vi "CreateLocalVI.vi"(10 "Name":string, 11 "YActor in":refnum<class "YActor.lvclass">) -> (3 "YActor out":refnum<class "YActor.lvclass">, 5 "CreatedVI":refnum<vi>)   [LabVIEW 2021, in "YActor.lvclass"]
uses:
  YActor.lvclass
  InlineReferencePool.ctl
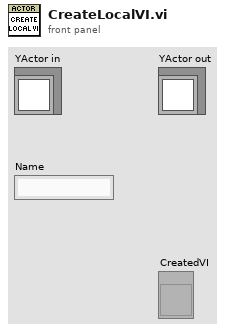
[diagram p1: front panel]
types:
  T1 = typedef "YActor.lvclass/InlineReferencePool.ctl" = enum16{"Add", "ClearAll?"}
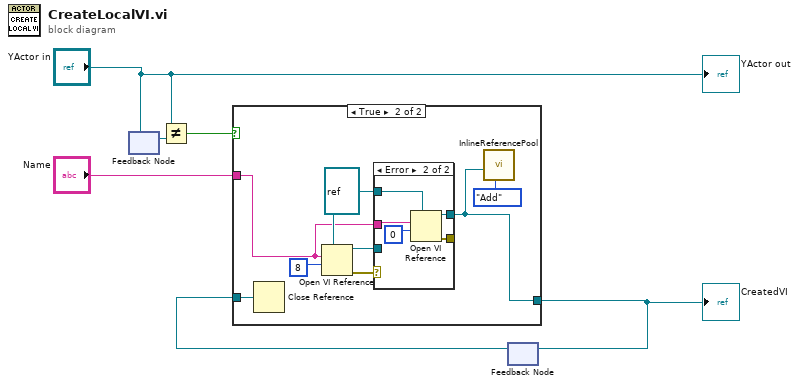
[diagram p0: block diagram]
diagram:
  n1 = feedback #1() -> (w5:refnum<class "YActor.lvclass">)  [unwired: 1 in]
  n2 = feedback-in #1("YActor in") -> ()
  n3 = Not Equal?(x="YActor in", y=w5) -> (x != y?=w6:bool)
  n4 = feedback #2() -> (w4:refnum<vi>)  [unwired: 1 in]
  n5 = case shown="True" w6 {
    tunnel: [w7 w9] -> w2
    tunnel: w4 -> [w7 w8]
    tunnel: "Name" -> [_ w11]
    frame False {
    }
    frame True {
      w14 = refnum<vi> refnum ("type specifier VI Refnum (for type only)")
      n6 = Close Reference(reference=w8) -> ()  [unwired: 1 in, 1 out]
      n7 = Open VI Reference(type specifier VI Refnum (for type only)=w14, vi path=w11, options=8) -> (vi reference=w13:refnum<vi>, error out=w15:errorcluster)  [unwired: 3 in]
      n8 = case shown="Error" w15 {
        selector: w15 -> [w17 _]
        tunnel: w11 -> [_ w21]
        tunnel: w14 -> [_ w20]
        tunnel: [w16 w19] -> w9
        tunnel: [w17 w22] -> _
        tunnel: w13 -> [w16 _]
        frame No Error {
        }
        frame Error {
          n9 = Open VI Reference(type specifier VI Refnum (for type only)=w20, vi path=w21, options=0) -> (vi reference=w19:refnum<vi>, error out=w22:errorcluster)  [unwired: 3 in]
        }
      }
      n10 = call "InlineReferencePool.vi"("functions"=InlineReferencePool."Add", "inline vi ref"=w9) -> ()  [unwired: 8 in, 2 out]
    }
  }
  "CreatedVI" <- w2
  n11 = feedback-in #2(w2) -> ()
  "YActor out" <- "YActor in"
